vi "RichToFlathwval_GenericResponse.vi"(5 "OutputClusterType":T1, 11 "InputCluster":T2) -> (3 "OutputCluster":T1)   [LabVIEW 2025, in "Automotive-Vision-OOBService_client.lvlib"]
uses:
  hwval_GenericResponse.ctl
  hwval_GenericResponse_Flat.ctl
  Automotive-Vision-OOBService_client.lvlib
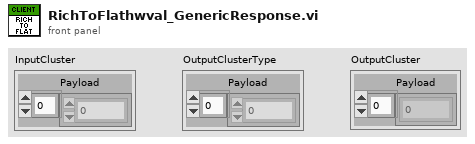
[diagram p1: front panel]
types:
  T1 = typedef "Automotive-Vision-OOBService_client.lvlib/hwval_GenericResponse_Flat.ctl" = cluster{"Payload":u8[]}
  T2 = typedef "Automotive-Vision-OOBService_client.lvlib/hwval_GenericResponse.ctl" = cluster{"Payload":u8[]}
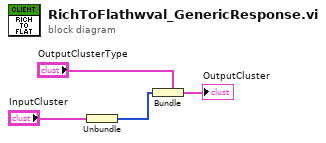
[diagram p0: block diagram]
diagram:
  n1 = Unbundle "Unbundle"("InputCluster") -> ("Payload"=w1:u8[])
  n2 = Bundle "Bundle"(cluster="OutputClusterType", "Payload"=w1) -> (→"OutputCluster":T1)
